vi "Not Equal (T).vi"(1 "Variant":variant) -> (0 "Changed":bool)   [LabVIEW 2017, in "Endigit.lvlib"]
doc: "Outputs true if the value of \"Variant\" is different from the last time this reentrant VI was called. Outputs a true the first time it is run.\n\nAuthored by Robert C. Mortensen\nrobert@endigit.com\n\nCopyright (c) 2015, Endigit, Inc."
uses:
  Endigit.lvlib
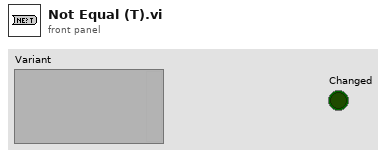
[diagram p1: front panel]
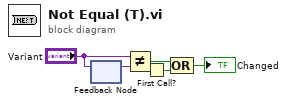
[diagram p0: block diagram]
diagram:
  n1 = feedback-in #1("Variant") -> ()
  n2 = feedback #1() -> (w5:variant)  [unwired: 1 in]
  n3 = Not Equal?(x="Variant", y=w5) -> (x != y?=w3:bool)
  n4 = First Call?() -> (First Call?: T/F=w2:bool)
  n5 = Compound Arithmetic op=OR(w3, w2) -> (→"Changed":bool)
